vi "Module Loop.vi"(8 "error in (no error)":errorcluster, 11 "DAQmxDI in":refnum<class "DAQmxDI.lvclass">) -> (0 "error out":errorcluster, 3 "DAQmxDI out":refnum<class "DAQmxDI.lvclass">)   [LabVIEW 2023, in "VolatusDAQ.lvlib" / "DAQmxDI.lvclass"]
uses:
  DAQmxDI.lvclass
  DAQmxDI.lvclass/DAQmxDI.ctl
  Volatus/Module/Module.lvclass/Module.ctl
  Volatus/MessageQ/MessageQ.lvclass/MessageQ.ctl
  Volatus/Module/Module.lvclass
  <vilib>/Utility/error.llb/Error Cluster From Error Code.vi
  Volatus/MessageQ/MessageQ.lvclass
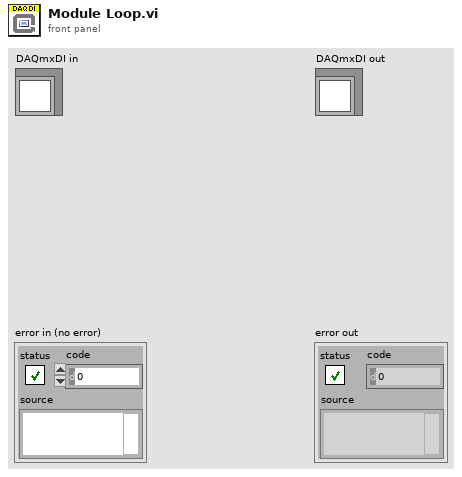
[diagram p1: front panel]
types:
  T1 = enum32{"Invalid", "Standard", "Closed", "Hidden", "Minimized", "Maximized"}
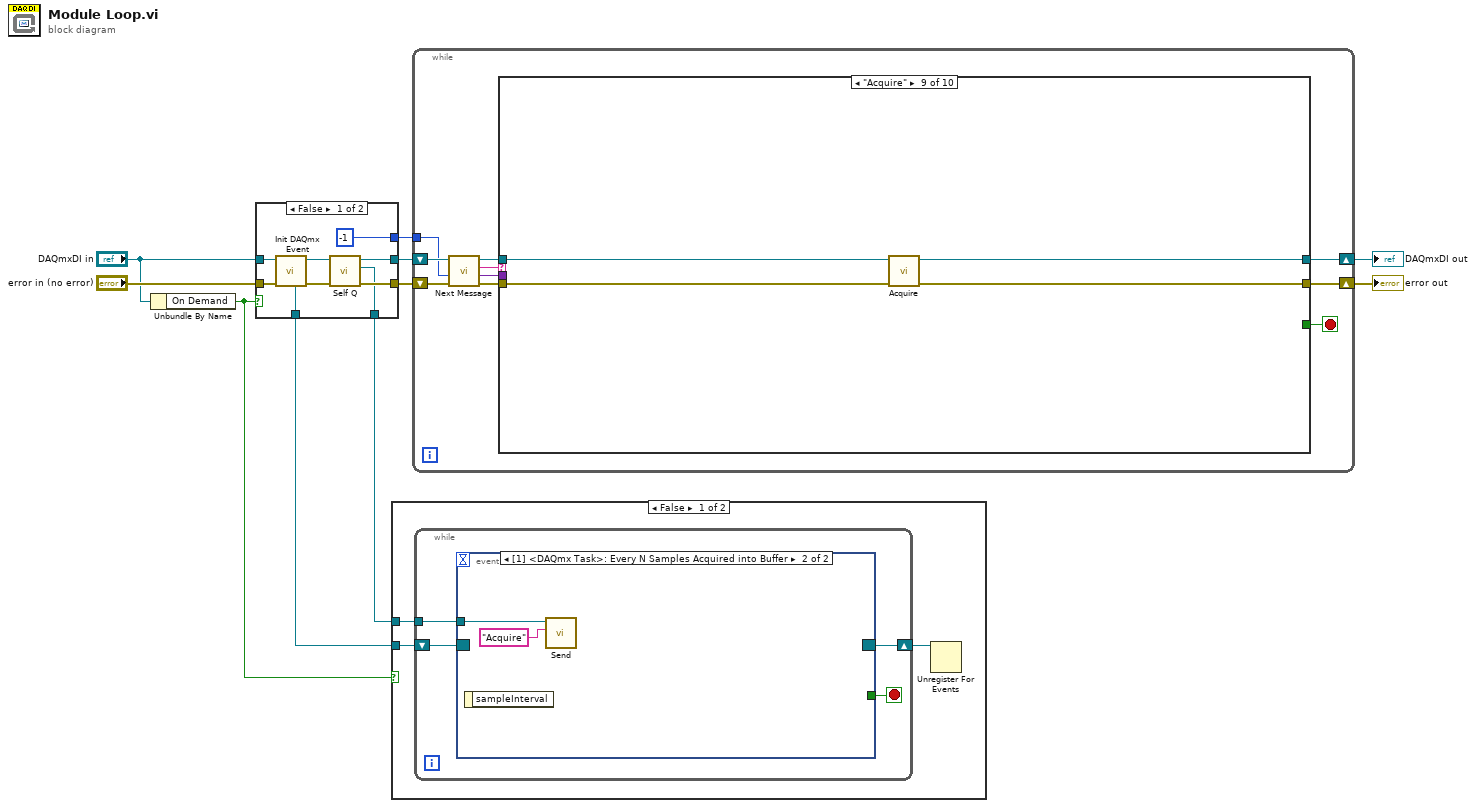
[diagram p0: block diagram]
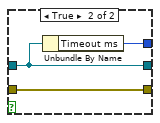
[diagram p2: hidden frame]
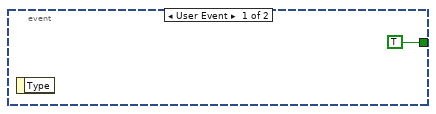
[diagram p3: hidden frame]
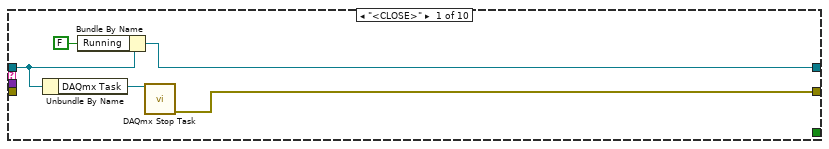
[diagram p5: hidden frame]
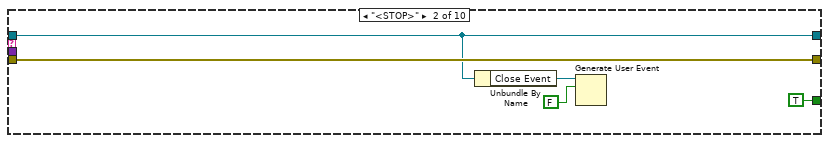
[diagram p6: hidden frame]
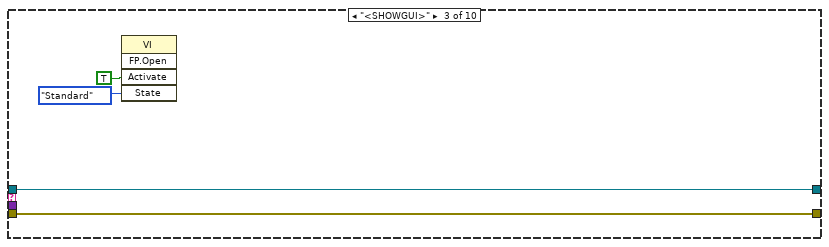
[diagram p7: hidden frame]
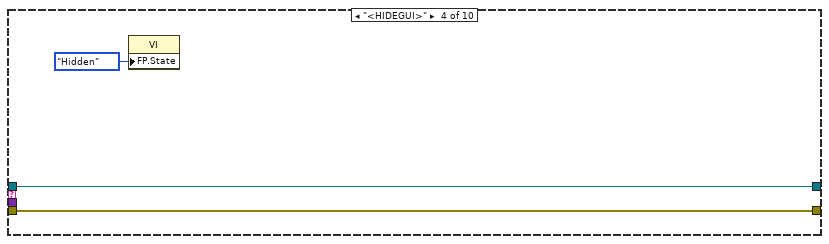
[diagram p8: hidden frame]
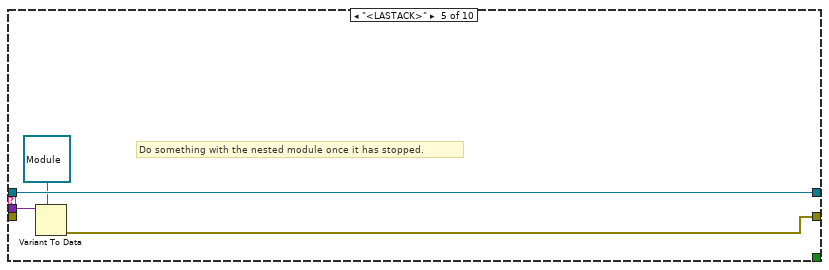
[diagram p9: hidden frame]
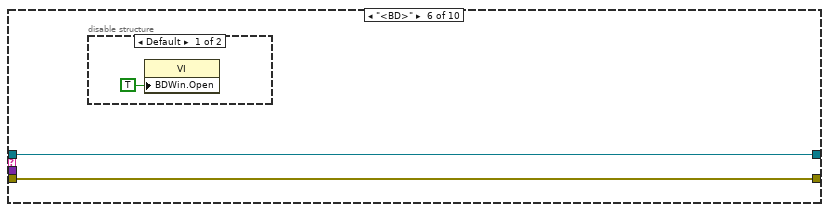
[diagram p10: hidden frame]
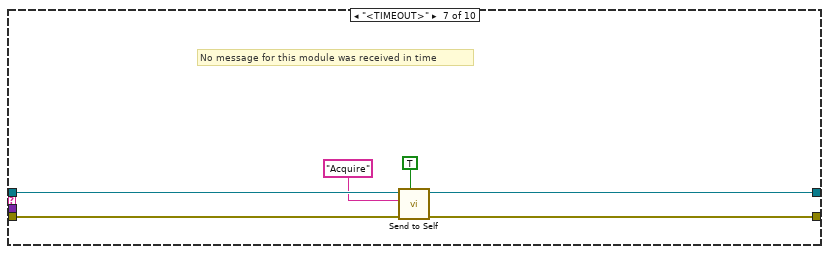
[diagram p12: hidden frame]
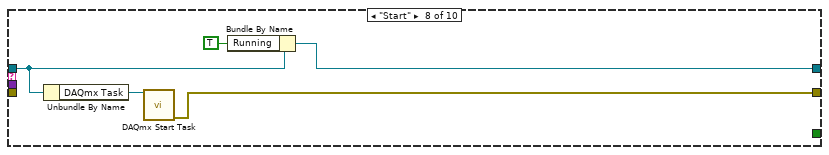
[diagram p13: hidden frame]
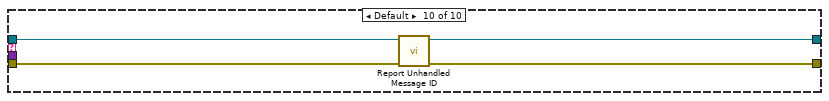
[diagram p14: hidden frame]
diagram:
  n1 = Unbundle By Name("DAQmxDI in") -> ("On Demand"=w1:bool)
  n2 = case shown="False" w1 {
    tunnel: "error in (no error)" -> [w18 w19]
    tunnel: [w17 w19] -> w7
    tunnel: "DAQmxDI in" -> [w16 w20]
    tunnel: [w14 _] -> w6
    tunnel: [w13 w20] -> w5
    tunnel: [w12 _] -> w4
    tunnel: [-1 ("Timeout/Period ms (-1)") w21] -> w2
    frame False {
      n3 = call "Init DAQmx Event.vi"("error in (no error)"=w18, "DAQmxDI in"=w16) -> ("error out"=w17:errorcluster, "DAQmxDI out"=w15:refnum<class "DAQmxDI.lvclass">, "Event Reg"=w14:refnum<event-registration>)  [unwired: 7 in]
      n4 = call "Self Q.vi"("Module in"=w15) -> ("Self Q"=w12:refnum<class "MessageQ.lvclass">, "Module out"=w13:refnum<class "DAQmxDI.lvclass">)  [unwired: 9 in]
    }
    frame True {
      n5 = Unbundle By Name(w20) -> ("Timeout ms"=w21:i32)
    }
  }
  n6 = case shown="False" w1 {
    tunnel: w6 -> [w23 _]
    tunnel: w4 -> [w22 _]
    frame False {
      n7 = while {
        tunnel: w22 -> [w27]
        shift-right: [w26] -> w24
        shift-left: w23 -> [w28]
        stop <- w25 stop-if-true
        n8 = event shown="[1] <DAQmx Task>: Every N Samples Acquired into Buffer" {
          selector: w28 -> [_ _]
          dyn-events: [_ _] -> w26
          timeout: _ -> [_ _]
          tunnel: w27 -> [_ w31]
          tunnel: [TRUE _] -> w25
          event User Event {
            n9 = event-data() -> ()  [unwired: 1 in, 1 out]
          }
          event Every N Samples Acquired into Buffer {
            n10 = event-data() -> ()  [unwired: 1 in, 1 out]
            n11 = call "Send.vi"("ID"="Acquire", "MessageQ in"=w31) -> ()  [unwired: 8 in, 2 out]
          }
        }
      }
      n12 = Unregister For Events(event registration refnum=w24) -> ()  [unwired: 1 in, 1 out]
    }
    frame True {
    }
  }
  n13 = while {
    shift-right: [w36] -> w9
    shift-left: w5 -> [w41]
    shift-right: [w35] -> w8
    shift-left: w7 -> [w40]
    tunnel: w2 -> [w32]
    stop <- w34 stop-if-true
    n14 = call "Next Message.vi"("error in (no error)"=w40, "Timeout/Period ms (-1)"=w32, "Module in"=w41) -> ("error out"=w39:errorcluster, "Data"=w33:variant, "ID"=w38:string, "Module out"=w37:refnum<class "DAQmxDI.lvclass">)  [unwired: 5 in]
    n15 = case shown="\"Acquire\"" w38 {
      tunnel: w39 -> [_ w51 w54 w57 _ w63 w71 _ w80 w84]
      tunnel: w37 -> [w45 w49 w55 w58 w62 w64 w69 w76 w78 w82]
      tunnel: [w43 w49 w55 w58 w62 w64 w68 w73 w77 w81] -> w36
      tunnel: [w44 w51 w54 w57 w59 w63 w70 w74 w79 w83] -> w35
      tunnel: [_ TRUE _ _ _ _ _ _ _ _] -> w34
      tunnel: w33 -> [_ _ _ _ w61 _ _ _ _ _]
      frame "<CLOSE>" {
        n16 = Unbundle By Name(w45) -> ("DAQmx Task"=w46:refnum<k21>)
        n17 = Bundle By Name(cluster=w45, "Running"=FALSE) -> (w43:refnum<class "DAQmxDI.lvclass">)
        n18 = call <vilib>:"DAQmx Stop Task.vi"("task/channels in"=w46) -> ("error out"=w44:errorcluster)  [unwired: 13 in, 1 out]
      }
      frame "<STOP>" {
        n19 = Unbundle By Name(w49) -> ("Close Event"=w48:refnum<user-event>)
        n20 = Generate User Event(user event=w48, event data cluster=FALSE ("event data")) -> ()  [unwired: 2 in, 2 out]
      }
      frame "<SHOWGUI>" {
        n21 = invoke class="VI" method="FP.Open"("Activate"=TRUE ("Activate?"), "State"=T1."Standard") -> ()  [unwired: 3 in, 5 out]
      }
      frame "<HIDEGUI>" {
        n22 = property class="VI"("FP.State"=T1."Hidden" ("Front Panel Window:State")) -> ()  [unwired: 2 in, 2 out]
      }
      frame "<LASTACK>" {
        # "Do something with the nested module once it has stopped."
        n23 = Variant To Data(type=refnum<class "Module.lvclass"> refnum ("Volatus:Module"), Variant=w61) -> (error out=w59:errorcluster)  [unwired: 1 in, 1 out]
      }
      frame "<BD>" {
        n24 = disable-structure shown="Default" {
          frame condition #0 (active) {
            n25 = property class="VI"("BDWin.Open"=TRUE ("Block Diagram Window:Open")) -> ()  [unwired: 2 in, 2 out]
          }
          frame condition #1 {
          }
        }
      }
      frame "<TIMEOUT>" {
        # "No message for this module was received in time"
        n26 = call "Send to Self.vi"("High Priority (F)"=TRUE, "error in (no error)"=w71, "Message ID"="Acquire", "Module in"=w69) -> ("error out"=w70:errorcluster, "Module out"=w68:refnum<class "DAQmxDI.lvclass">)  [unwired: 6 in]
      }
      frame "Start" {
        n27 = Unbundle By Name(w76) -> ("DAQmx Task"=w75:refnum<k21>)
        n28 = call <vilib>:"DAQmx Start Task.vi"("task/channels in"=w75) -> ("error out"=w74:errorcluster)  [unwired: 13 in, 1 out]
        n29 = Bundle By Name(cluster=w76, "Running"=TRUE) -> (w73:refnum<class "DAQmxDI.lvclass">)
      }
      frame "Acquire" {
        n30 = call "Acquire.vi"("error in (no error)"=w80, "DAQmxDI in"=w78) -> ("error out"=w79:errorcluster, "DAQmxDI out"=w77:refnum<class "DAQmxDI.lvclass">)  [unwired: 8 in]
      }
      frame Default {
        n31 = call "Report Unhandled Message ID.vi"("error in (no error)"=w84, "Module in"=w82) -> ("error out"=w83:errorcluster, "Module out"=w81:refnum<class "DAQmxDI.lvclass">)  [unwired: 8 in]
      }
    }
  }
  "error out" <- w8
  "DAQmxDI out" <- w9
